vi "Herdsimulation.vi"() -> ()   [LabVIEW 2019]
panel:
  out "Test":dbl
  out "Soll Temperatur":u8
  in  "Stopp":bool
  out "Heizspule aktiv":bool
  out "Temperatur":u8
  out "Signalverlaufsdiagramm":u8[][](graph)
  in  "Drehregler":u8(knob) max=3 step=1 scale=0.0..3.0
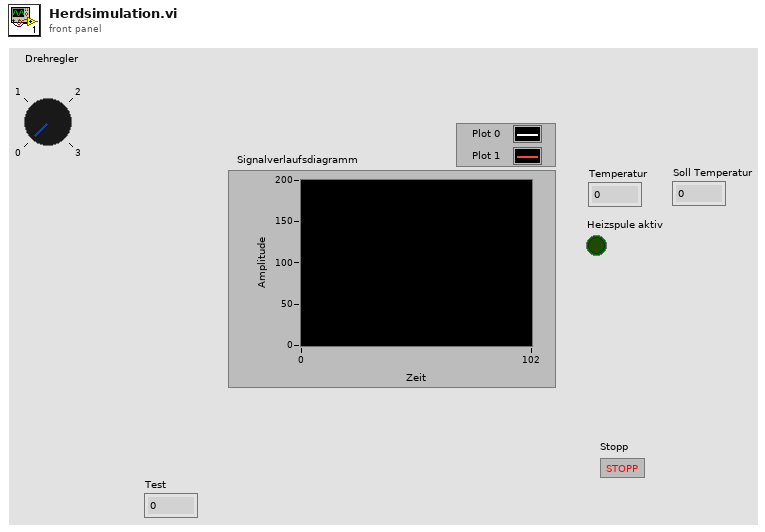
[diagram p1: front panel]
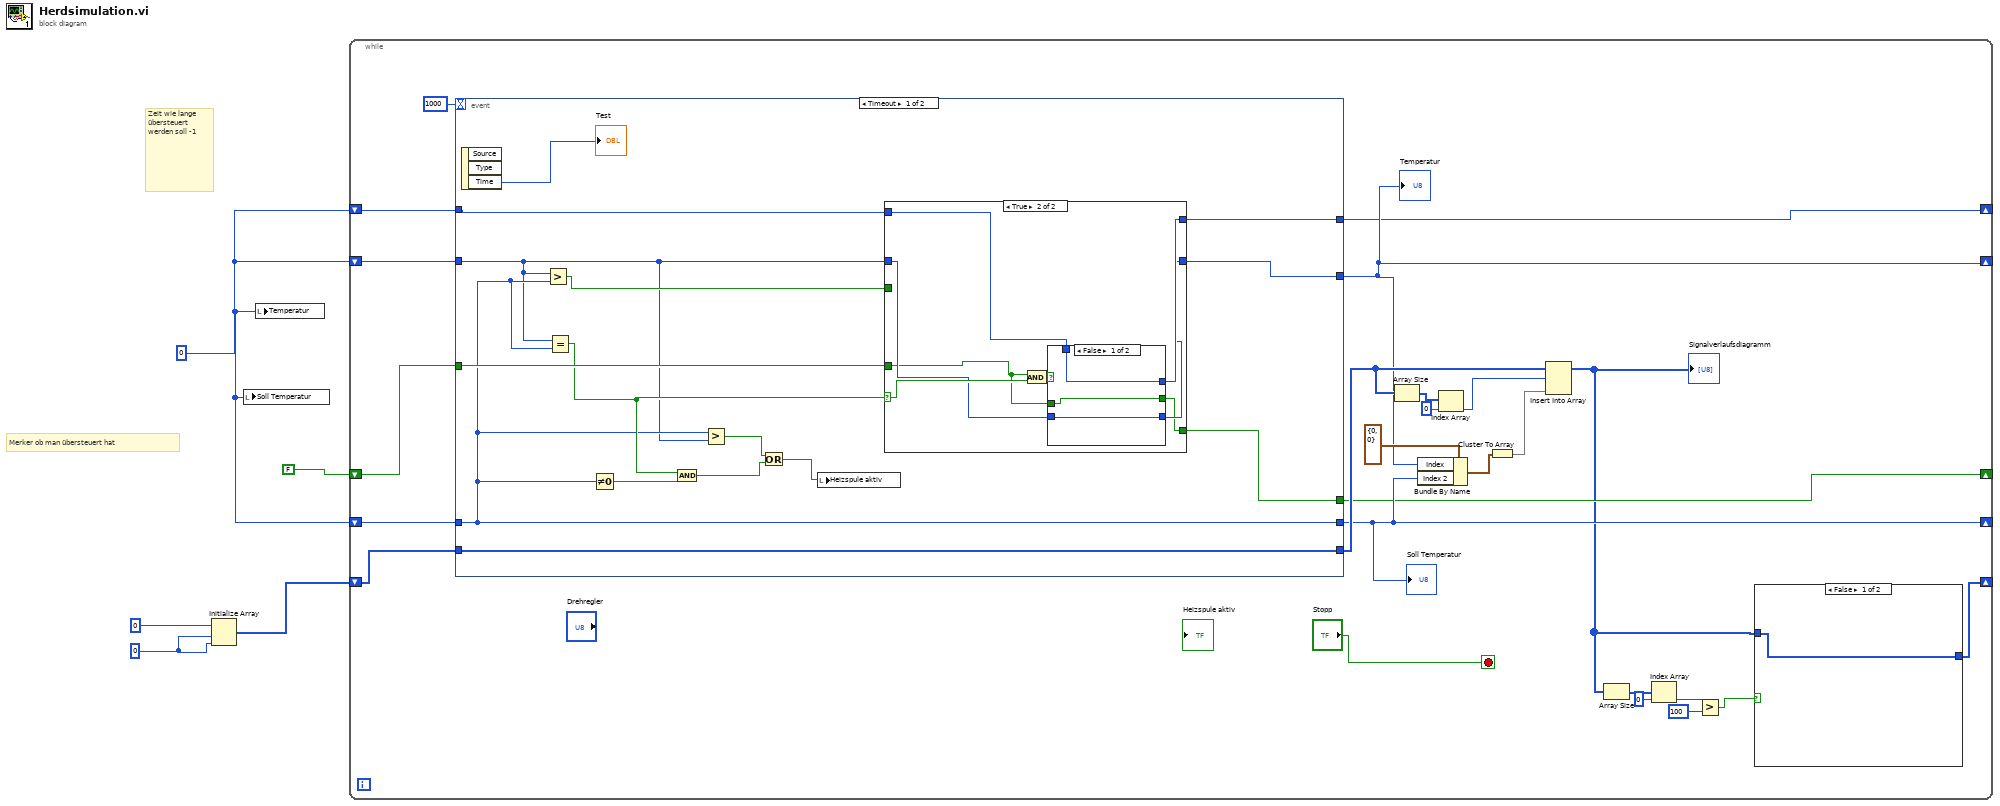
[diagram p0: block diagram]
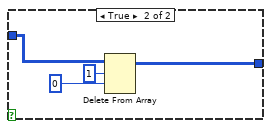
[diagram p2: hidden frame]
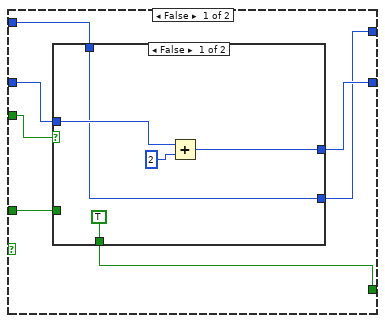
[diagram p3: hidden frame]
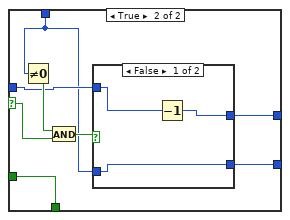
[diagram p4: hidden frame]
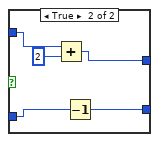
[diagram p5: hidden frame]
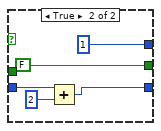
[diagram p6: hidden frame]
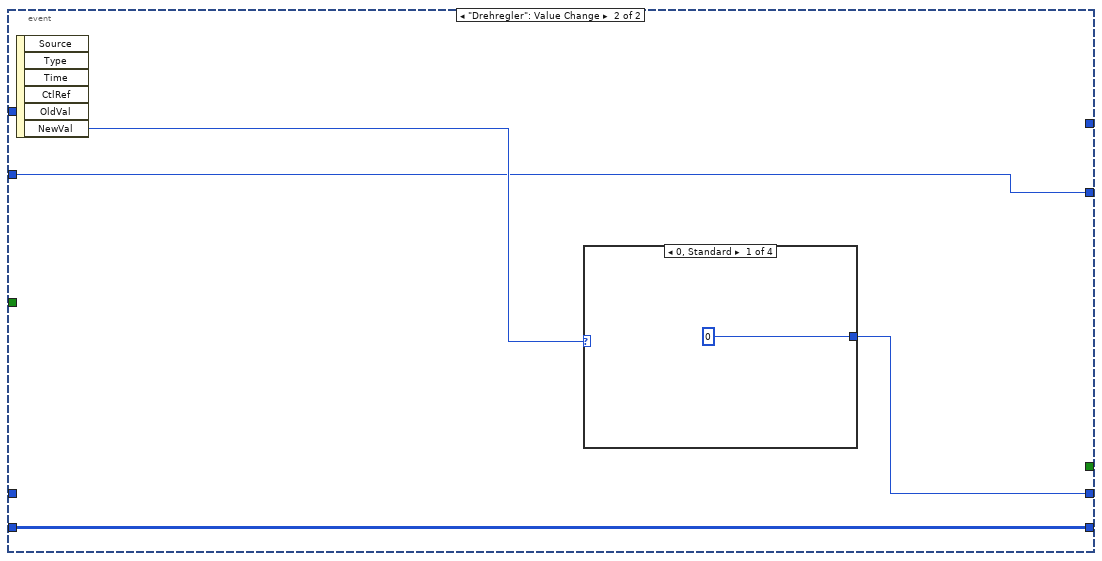
[diagram p7: hidden frame]
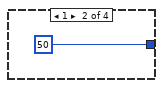
[diagram p8: hidden frame]
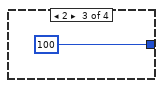
[diagram p9: hidden frame]
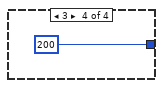
[diagram p10: hidden frame]
diagram:
  w5 = 0
  w2 = u8 0 ("Temperatur")
  # "Zeit wie lange übersteuert werden soll -1"
  # "Merker ob man übersteuert hat"
  n1 = Initialize Array(u8 0, w5, w5) -> (w4:u8[][])
  n2 = local write "Soll Temperatur"(w2) -> ()
  n3 = local write "Temperatur"(w2) -> ()
  n4 = while {
    shift-right: [w18] -> _
    shift-left: w2 -> [w30]
    shift-right: [w17] -> _
    shift-left: w2 -> [w29]
    shift-right: [w6] -> _
    shift-left: w4 -> [w26]
    shift-right: [w15] -> _
    shift-left: w2 -> [w16]
    shift-right: [w13] -> _
    shift-left: FALSE -> [w14]
    stop <- "Stopp" stop-if-true
    n5 = event shown="[0] Timeout" {
      selector: _ -> [_ _]
      dyn-events: _ -> [_ _]
      timeout: 1000 -> [_ _]
      tunnel: w30 -> [w37 _]
      tunnel: [w37 w97] -> w18
      tunnel: w29 -> [w36 w95]
      tunnel: [w48 w95] -> w17
      tunnel: w26 -> [w49 w96]
      tunnel: [w49 w96] -> w25
      tunnel: w16 -> [w47 _]
      tunnel: [w46 _] -> w15
      tunnel: w14 -> [w42 _]
      tunnel: [w45 _] -> w13
      event Timeout {
        n6 = event-data() -> ("Time"=→"Test":u32)  [unwired: 1 in, 2 out]
        n7 = Greater?(x=w36, y=w37) -> (0:w44:bool)
        n8 = Equal?(x=w36, y=w37) -> (x = y?=w41:bool)
        n9 = Not Equal To 0?(x=w37) -> (x != 0?=w40:bool)
        n10 = And(x=w41, y=w40) -> (x .and. y?=w39:bool)
        n11 = Greater?(x=w37, y=w36) -> (0:w38:bool)
        n12 = Or(x=w38, y=w39) -> (x .or. y?=w43:bool)
        n13 = local write "Heizspule aktiv"(w43) -> ()
        n14 = case shown="True" w41 {
          selector: w41 -> [_ w86]
          tunnel: w36 -> [w57 w82]
          tunnel: w44 -> [w55 _]
          tunnel: [w56 w81] -> w48
          tunnel: w47 -> [w54 w83]
          tunnel: [w53 w84] -> w46
          tunnel: w42 -> [w52 w79]
          tunnel: [w51 w80] -> w45
          frame False {
            n15 = case shown="False" w55 {
              selector: w55 -> [_ w68]
              tunnel: w57 -> [w62 w67]
              tunnel: [w60 w66] -> w56
              tunnel: w54 -> [w59 w65]
              tunnel: [w59 w64] -> w53
              tunnel: w52 -> [_ w63]
              tunnel: [TRUE ("Heizspule aktiv") w63] -> w51
              frame False {
                n16 = Add(x=w62, y=u8 2) -> (x+y=w60:u8)
              }
              frame True {
                n17 = Not Equal To 0?(x=w65) -> (x != 0?=w69:bool)
                n18 = And(x=w69, y=w68) -> (x .and. y?=w70:bool)
                n19 = case shown="False" w70 {
                  tunnel: w67 -> [w72 w76]
                  tunnel: [w73 w75] -> w66
                  tunnel: w65 -> [w71 w78]
                  tunnel: [w71 w77] -> w64
                  frame False {
                    n20 = Decrement(x=w72) -> (x-1=w73:u8)
                  }
                  frame True {
                    n21 = Add(x=w76, y=u8 2) -> (x+y=w75:u8)
                    n22 = Decrement(x=w78) -> (x-1=w77:u8)
                  }
                }
              }
            }
          }
          frame True {
            n23 = And(x=w79, y=w86) -> (x .and. y?=w85:bool)
            n24 = case shown="False" w85 {
              tunnel: [w89 u8 1] -> w84
              tunnel: w83 -> [w89 _]
              tunnel: w82 -> [w88 w93]
              tunnel: [w88 w92] -> w81
              tunnel: [w87 FALSE ("Heizspule aktiv")] -> w80
              tunnel: w79 -> [w87 _]
              frame False {
              }
              frame True {
                n25 = Add(x=w93, y=u8 2) -> (x+y=w92:u8)
              }
            }
          }
        }
      }
      event "Drehregler": Value Change {
        n26 = event-data() -> ("NewVal"=w98:u8)  [unwired: 1 in, 5 out]
        n27 = case shown="0, Standard" w98 {
          tunnel: [u8 0 u8 50 u8 100 u8 200] -> w97
          frame 0, Default {
          }
          frame 1 {
          }
          frame 2 {
          }
          frame 3 {
          }
        }
      }
    }
    "Temperatur" <- w17
    "Soll Temperatur" <- w18
    n28 = Array Size(array=w25) -> (size(s)=w24:i32[])
    n29 = Bundle By Name(cluster=cluster{"Index":u8, "Index 2":u8} {"Index"=0, "Index 2"=0}, "Index"=w17, "Index 2"=w18) -> (w19:cluster{"Index":u8, "Index 2":u8})
    n30 = Index Array(array=w24, index=0 ("Index")) -> (element=w22:i32)
    n31 = Cluster To Array(cluster=w19) -> (array=w21:u8[])
    n32 = Insert Into Array(array=w25, index (row)=w22, new element=w21) -> (w7:u8[][])  [unwired: 1 in]
    "Signalverlaufsdiagramm" <- w7
    n33 = Array Size(array=w7) -> (size(s)=w12:i32[])
    n34 = Index Array(array=w12, index=0 ("Index")) -> (element=w10:i32)
    n35 = Greater?(x=w10, y=100) -> (0:w8:bool)
    n36 = case shown="False" w8 {
      tunnel: w7 -> [w31 w35]
      tunnel: [w31 w32] -> w6
      frame False {
      }
      frame True {
        n37 = Delete From Array(array=w35, length=1 ("Länge"), index (row)=0 ("Index (Zeile)")) -> (array with subset deleted=w32:u8[][])  [unwired: 1 in, 1 out]
      }
    }
  }
